vi "Get-Available-filter-types.vi"(8 "error in":errorcluster, 10 "Temp. params. ref.":refnum<data-value>, 11 "Analysis params. ref.":refnum<data-value>) -> (0 "error IO":errorcluster, 1 "Available filters":T1[](array[typedef]))   [LabVIEW 2013, in "CameraVision.lvlib" / "CV-Filter.lvclass"]
uses:
  CV-Filter.lvclass
  Filter-characteristic.ctl
  Temperature/CV-Temperature.lvclass
  Analysis/CV-Analysis.lvclass
  Temperature/CV-Temperature.lvclass/CV-Temperature.ctl
  Analysis/CV-Analysis.lvclass/CV-Analysis.ctl
  Analysis/Read Image characteristics.vi
  Analysis/Read Melt-pool characteristics.vi
  Temperature/Read Temperature value.vi
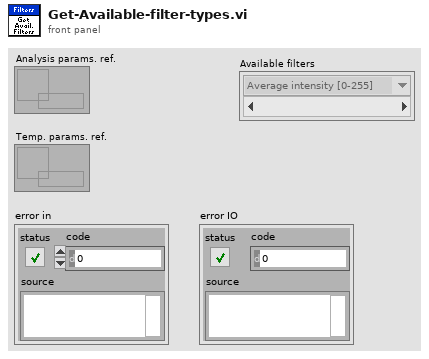
[diagram p1: front panel]
types:
  T1 = typedef "CameraVision.lvlib/CV-Filter.lvclass/Filter-characteristic.ctl" = enum16{"Average intensity [0-255]", "Peak intensity [0-255]", "Melt-pool size [mm²]", "Melt-pool aspect ratio []", "Melt-pool fragments []", "Melt-pool position X [pixel]", "Melt-pool position Y [pixel]", "Average temperature [°C]", "Max. temperature [°C]", "Min. temperature [°C]", "Std. dev. temperature [°C]"}
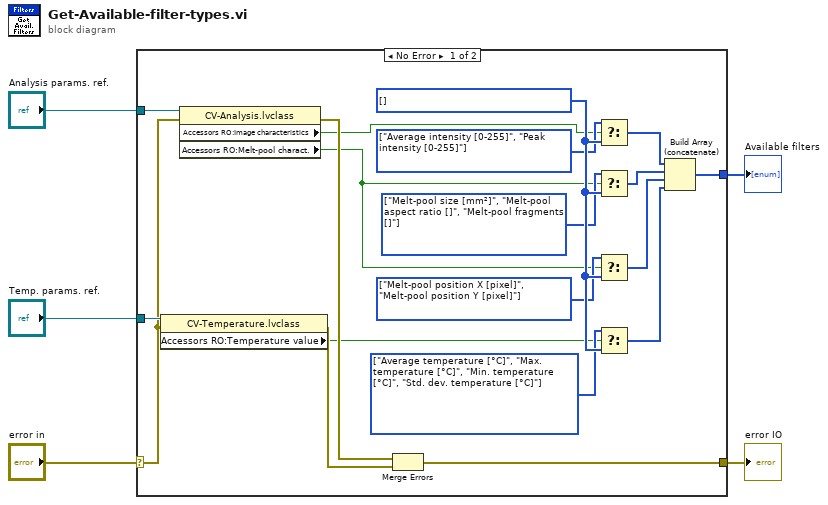
[diagram p0: block diagram]
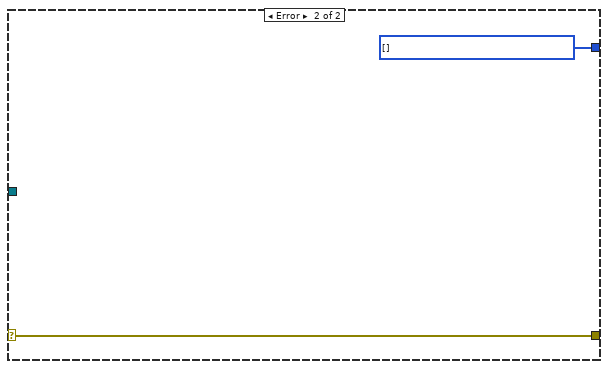
[diagram p2: hidden frame]
diagram:
  n1 = case shown="No Error" "error in" {
    selector: "error in" -> [w7 w26]
    tunnel: [w24 w26] -> w5
    tunnel: [w23 w25] -> w4
    tunnel: "Temp. params. ref." -> [w9 _]
    tunnel: "Analysis params. ref." -> [w8 _]
    frame No Error {
      w13 = T1[] [enum."Melt-pool position X [pixel]", enum."Melt-pool position Y [pixel]"] items=["Average intensity [0-255]", "Peak intensity [0-255]", "Melt-pool size [mm²]", "Melt-pool aspect ratio []", "Melt-pool fragments []", "Melt-pool position X [pixel]", "Melt-pool position Y [pixel]", "Average temperature [°C]", "Max. temperature [°C]", "Min. temperature [°C]", "Std. dev. temperature [°C]"]
      w12 = T1[] [enum."Average temperature [°C]", enum."Max. temperature [°C]", enum."Min. temperature [°C]", enum."Std. dev. temperature [°C]"] items=["Average intensity [0-255]", "Peak intensity [0-255]", "Melt-pool size [mm²]", "Melt-pool aspect ratio []", "Melt-pool fragments []", "Melt-pool position X [pixel]", "Melt-pool position Y [pixel]", "Average temperature [°C]", "Max. temperature [°C]", "Min. temperature [°C]", "Std. dev. temperature [°C]"]
      w14 = T1[] [enum."Melt-pool size [mm²]", enum."Melt-pool aspect ratio []", enum."Melt-pool fragments []"] items=["Average intensity [0-255]", "Peak intensity [0-255]", "Melt-pool size [mm²]", "Melt-pool aspect ratio []", "Melt-pool fragments []", "Melt-pool position X [pixel]", "Melt-pool position Y [pixel]", "Average temperature [°C]", "Max. temperature [°C]", "Min. temperature [°C]", "Std. dev. temperature [°C]"]
      w15 = T1[] [enum."Average intensity [0-255]", enum."Peak intensity [0-255]"] items=["Average intensity [0-255]", "Peak intensity [0-255]", "Melt-pool size [mm²]", "Melt-pool aspect ratio []", "Melt-pool fragments []", "Melt-pool position X [pixel]", "Melt-pool position Y [pixel]", "Average temperature [°C]", "Max. temperature [°C]", "Min. temperature [°C]", "Std. dev. temperature [°C]"]
      w16 = T1[] [] items=["Average intensity [0-255]", "Peak intensity [0-255]", "Melt-pool size [mm²]", "Melt-pool aspect ratio []", "Melt-pool fragments []", "Melt-pool position X [pixel]", "Melt-pool position Y [pixel]", "Average temperature [°C]", "Max. temperature [°C]", "Min. temperature [°C]", "Std. dev. temperature [°C]"]
      n2 = property class="CV-Temperature.lvclass"(reference=w9, error in=w7) -> (error out=w22:errorcluster, "Accessors RO:Temperature value"=w11:bool)  [unwired: 1 out]
      n3 = property class="CV-Analysis.lvclass"(reference=w8, error in=w7) -> (error out=w21:errorcluster, "Accessors RO:Image characteristics"=w10:bool, "Accessors RO:Melt-pool charact."=w6:bool)  [unwired: 1 out]
      n4 = Merge Errors(w21, w22) -> (w24:errorcluster)
      n5 = Select(t=w15, s=w10, f=w16) -> (s? t:f=w17:T1[])
      n6 = Select(t=w14, s=w6, f=w16) -> (s? t:f=w18:T1[])
      n7 = Select(t=w13, s=w6, f=w16) -> (s? t:f=w20:T1[])
      n8 = Select(t=w12, s=w11, f=w16) -> (s? t:f=w19:T1[])
      n9 = Build Array (concatenate)(w17, w18, w20, w19) -> (w23:T1[])
    }
    frame Error {
      w25 = T1[] [] items=["Average intensity [0-255]", "Peak intensity [0-255]", "Melt-pool size [mm²]", "Melt-pool aspect ratio []", "Melt-pool fragments []", "Melt-pool position X [pixel]", "Melt-pool position Y [pixel]", "Average temperature [°C]", "Max. temperature [°C]", "Min. temperature [°C]", "Std. dev. temperature [°C]"]
    }
  }
  "error IO" <- w5
  "Available filters" <- w4
